vi "delete directory and contents.vi"(2 "error in":errorcluster, 3 "Directory to delete":path=path "\\\\Enviro\\enviro/Software/RunTime7") -> (0 "error out":errorcluster, 1 "dup directory path":path)   [LabVIEW 2010]
panel:
  out "Current file":string
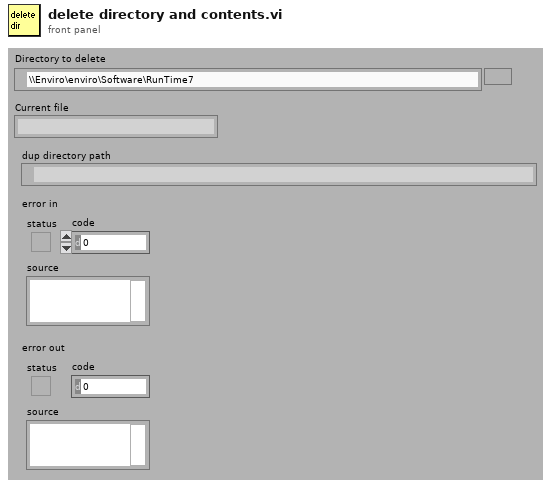
[diagram p1: front panel]
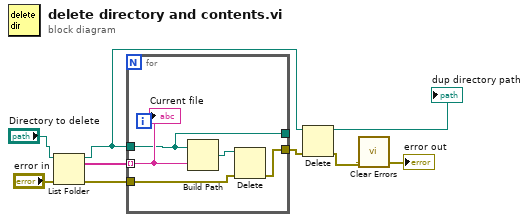
[diagram p0: block diagram]
diagram:
  n1 = List Folder(path="Directory to delete", error in="error in") -> (path out=w5:path, filenames=w7:string[], error out=w4:errorcluster)  [unwired: 2 in, 1 out]
  "dup directory path" <- w5
  n2 = for {
    tunnel: w5 -> [w11]
    tunnel: w7 -> [w12] mode=indexing
    tunnel: [w11] -> _
    tunnel: [w10] -> w6
    tunnel: w4 -> [w9]
    n3 = Build Path(base path=w11, name or relative path=w12) -> (appended path=w13:path)
    n4 = Delete(path (use dialog)=w13, error in=w9) -> (error out=w10:errorcluster)  [unwired: 3 in, 2 out]
    "Current file" <- w12
  }
  n5 = Delete(path (use dialog)=w5, error in=w6) -> (error out=w2:errorcluster)  [unwired: 3 in, 2 out]
  n6 = call <vilib>:"Clear Errors.vi"("error in (no error)"=w2) -> ("error out"=→"error out":errorcluster)  [unwired: 6 in]
